vi "Init Module.vi"(8 "error in":errorcluster, 11 "Singleton Module Admin in":refnum<class "Delacor_lib_QMH_Module Admin.lvclass">) -> (0 "error out":errorcluster, 1 "Panther Dashboard Broadcast Events":T1, 2 "Panther Dashboard Request Events":T2, 3 "Singleton Module Admin out":refnum<class "Delacor_lib_QMH_Module Admin.lvclass">)   [LabVIEW 2019, in "Panther Dashboard.lvlib"]
doc: "Initialize the module by creating Broadcast Events, Request Events, and synchronization rendezvous.\n_____\nBased on DQMH Project Template 6.1.0.94."
uses:
  Panther Dashboard.lvlib
  <vilib>/Delacor/Delacor QMH/Libraries/Module Admin_class/Delacor_lib_QMH_Module Admin.lvclass
  Request Events--cluster.ctl
  Stop Argument--cluster.ctl
  Show Panel Argument--cluster.ctl
  Hide Panel Argument--cluster.ctl
  Get Module Execution Status Argument--cluster.ctl
  Show Diagram Argument--cluster.ctl
  Scan DQMH Modules Argument--cluster.ctl
  Tree DQMH Selection Argument--cluster.ctl
  Open Module API Tester Argument--cluster.ctl
  Execute Default Event Request Argument--cluster.ctl
  Expand Results Argument--cluster.ctl
  Launch DQMH Scripting Tools Argument--cluster.ctl
  DQMH Tools Menu--enum.ctl
  Generate Project Documentation Argument--cluster.ctl
  Set App Theme Argument--cluster.ctl
  Show About Argument--cluster.ctl
  Update Module ID Argument--cluster.ctl
  Save Library Description Argument--cluster.ctl
  Save VI Description Argument--cluster.ctl
  Open Documentation Argument--cluster.ctl
  Set Pane Initial State Argument--cluster.ctl
  Broadcast Events--cluster.ctl
  Did Init Argument--cluster.ctl
  Status Updated Argument--cluster.ctl
  Error Reported Argument--cluster.ctl
  References Updated Argument--cluster.ctl
  Module type--enum.ctl
  Projects Updated Argument--cluster.ctl
  Targets Updated Argument--cluster.ctl
  Progress updated Argument--cluster.ctl
  Scale Updated Argument--cluster.ctl
  Connector Pane Updated Argument--cluster.ctl
  Documentation Updated Argument--cluster.ctl
  Documentation--cluster.ctl
  Module Type Updated Argument--cluster.ctl
  Theme Updated Argument--cluster.ctl
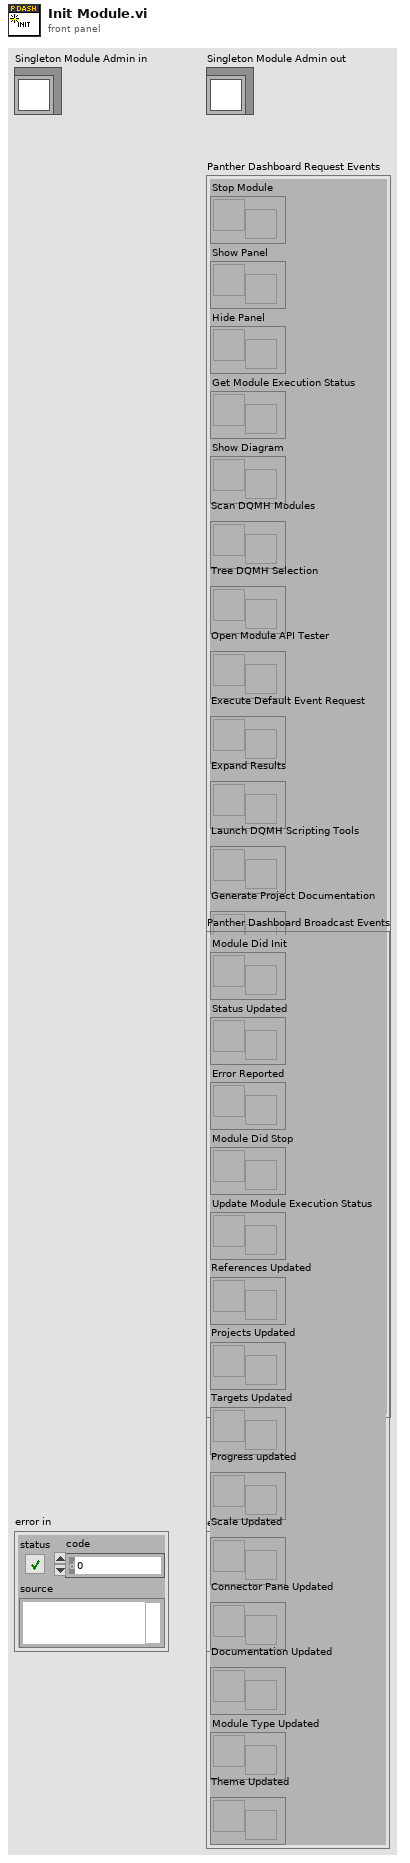
[diagram p1: front panel]
types:
  T1 = typedef "Panther Dashboard.lvlib/Broadcast Events--cluster.ctl" = cluster{"Module Did Init":refnum<user-event>, "Status Updated":refnum<user-event>, "Error Reported":refnum<user-event>, "Module Did Stop":refnum<user-event>, "Update Module Execution Status":refnum<user-event>, "References Updated":refnum<user-event>, "Projects Updated":refnum<user-event>, "Targets Updated":refnum<user-event>, "Progress updated":refnum<user-event>, "Scale Updated":refnum<user-event>, "Connector Pane Updated":refnum<user-event>, "Documentation Updated":refnum<user-event>, "Module Type Updated":refnum<user-event>, "Theme Updated":refnum<user-event>}
  T2 = typedef "Panther Dashboard.lvlib/Request Events--cluster.ctl" = cluster{"Stop Module":refnum<user-event>, "Show Panel":refnum<user-event>, "Hide Panel":refnum<user-event>, "Get Module Execution Status":refnum<user-event>, "Show Diagram":refnum<user-event>, "Scan DQMH Modules":refnum<user-event>, "Tree DQMH Selection":refnum<user-event>, "Open Module API Tester":refnum<user-event>, "Execute Default Event Request":refnum<user-event>, "Expand Results":refnum<user-event>, "Launch DQMH Scripting Tools":refnum<user-event>, "Generate Project Documentation":refnum<user-event>, "Set App Theme":refnum<user-event>, "Show About":refnum<user-event>, "Update Module ID":refnum<user-event>, "Save Library Description":refnum<user-event>, "Save VI Description":refnum<user-event>, "Open Documentation":refnum<user-event>, "Set Pane Initial State":refnum<user-event>}
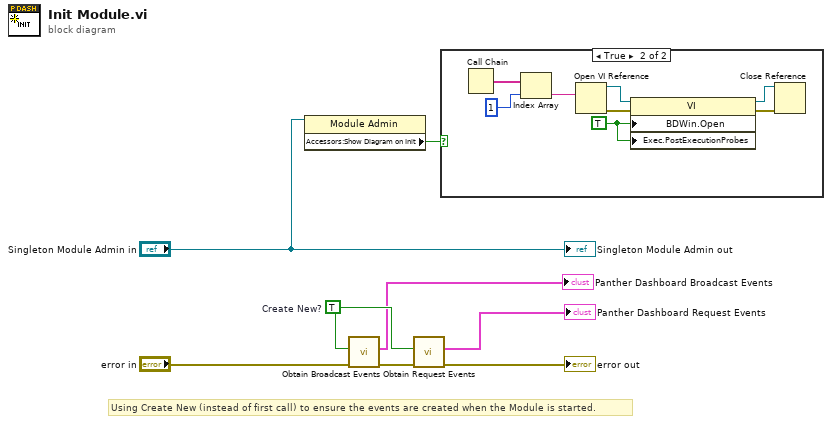
[diagram p0: block diagram]
diagram:
  w4 = TRUE  # Create New?
  # "Using Create New (instead of first call) to ensure the events are created when the Module is started."
  n1 = property class="Module Admin"(reference="Singleton Module Admin in") -> ("Accessors:Show Diagram on Init"=w3:bool)  [unwired: 1 in, 2 out]
  n2 = call "Obtain Broadcast Events.vi"("error in"="error in", "Create New? (F)"=w4) -> ("error out"=w8:errorcluster, "Panther Dashboard Broadcast Events"=→"Panther Dashboard Broadcast Events":T1)  [unwired: 8 in]
  n3 = call "Obtain Request Events.vi"("error in (no error)"=w8, "Create New? (F)"=w4) -> ("error out"=→"error out":errorcluster, "Panther Dashboard Request Events"=→"Panther Dashboard Request Events":T2)  [unwired: 8 in]
  n4 = case shown="True" w3 {
    frame False {
    }
    frame True {
      w11 = TRUE ("Block Diagram Window:Open")
      n5 = Call Chain() -> (call chain=w14:string[])
      n6 = Index Array(array=w14, index=1) -> (element=w9:string)
      n7 = Open VI Reference(vi path=w9) -> (vi reference=w12:refnum<vi>, error out=w16:errorcluster)  [unwired: 5 in]
      n8 = property class="VI"(reference=w12, error in=w16, "BDWin.Open"=w11, "Exec.PostExecutionProbes"=w11) -> (reference out=w10:refnum<vi>, error out=w15:errorcluster)
      n9 = Close Reference(reference=w10, error in (no error)=w15) -> ()  [unwired: 1 out]
    }
  }
  "Singleton Module Admin out" <- "Singleton Module Admin in"
